vi "System-AckFaults.vi"   [LabVIEW 2016, in "DSI-RT.lvlib"]
uses:
  DSI-RT.lvlib
  <vilib>/addons/Software Calibration Management/xSCM/FaultPoint.xnode
  <vilib>/addons/Software Calibration Management/xSCM/CalPoint.xnode
  <vilib>/addons/Software Calibration Management/xSCM/ni_scm.dll
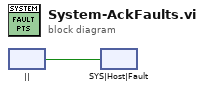
[diagram p0: block diagram]
diagram:
  n1 = xnode "||"() -> ("Fault"=w1:bool)
  n2 = xnode "SYS|Host|Fault"("Value"=w1) -> ()
